vi "Send Network Message.vi"(0 "message queue in":T2, 1 "receiver process":string, 2 "receiver host":string, 3 "receiver port (0)":u16, 5 "message name":string, 7 "message value":string, 9 "timeout (25000 ms)":i32=25000, 11 "error in":errorcluster, 12 "message attributes":T1, 13 "priority message (F)":bool, 14 "acknowledge message (F)":bool) -> (4 "message queue out":T2, 10 "timed out?":bool, 15 "error out":errorcluster)   [LabVIEW 2015, in "TLB` Template.lvlib" / "AMC.lvlib"]
doc: "Adds a message to the message dispatch queue in another application instance if the receiver host and process are specified. If the receiver host and process are undefined, or if they match the local application instance, then the message is added to the appropriate local message queue.\n\nIf \"receiver port\" is undefined, this VI will attempt to use the default UDP port.\n\nIf \"priority message\" is True, the message will be added to the front of the message queue.\n\nIf \"acknowledge message\" is True and the message is sent to another application instance, the receiver will send a reply message with the name format of \"AMC_Ack\" and a value of <name>. If \"message queue in\" is undefined, no acknowledge message will be sent.TLB Prime - Application Template 1.3.0.24\nNorm Kirchner, NI Systems Engineering - NI\nCopyright (c) 2014, NI"
uses:
  AMC.lvlib
  Message Queue.ctl
  Message.ctl
  Tools/Keyed Array/KeyedArray.ctl
  Tools/Keyed Array/Tools_KeyedArray.lvlib
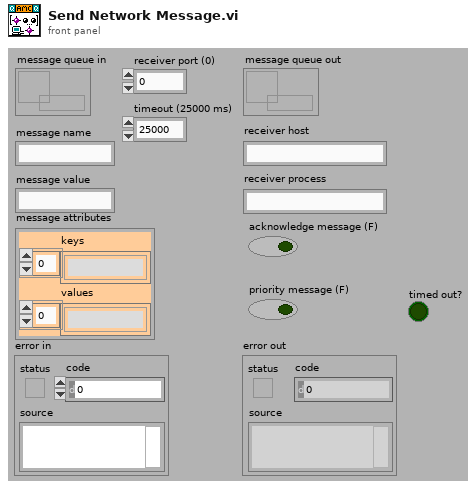
[diagram p1: front panel]
types:
  T1 = typedef "TLB` Template.lvlib/Tools_KeyedArray.lvlib/KeyedArray.ctl" = cluster{"keys":string[], "values":string[]}
  T2 = typedef "TLB` Template.lvlib/AMC.lvlib/Message Queue.ctl" = refnum<queue>
  T3 = typedef "TLB` Template.lvlib/AMC.lvlib/Message.ctl" = cluster{"name":string, "value":string, "attributes":T1, "receiver host":string, "receiver process":string, "source host":string, "source process":string, "priority message":bool, "acknowledge message":bool}
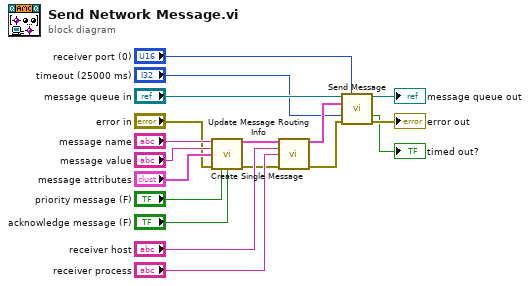
[diagram p0: block diagram]
diagram:
  n1 = call "Create Single Message.vi"("name"="message name", "value"="message value", "attributes"="message attributes", "error in"="error in", "priority message (F)"="priority message (F)", "acknowledge message (F)"="acknowledge message (F)") -> ("message"=w10:T3, "error out"=w6:errorcluster)  [unwired: 8 in]
  n2 = call "Update Message Routing Info.vi"("message"=w10, "receiver host (\"\")"="receiver host", "receiver process (\"\")"="receiver process", "error in"=w6) -> ("message"=w9:T3, "error out"=w5:errorcluster)  [unwired: 10 in]
  n3 = call "Send Message.vi"("message queue in"="message queue in", "receiver port (0)"="receiver port (0)", "message"=w9, "timeout (-1 ms)"="timeout (25000 ms)", "error in"=w5) -> ("message queue out"=→"message queue out":T2, "timed out?"=→"timed out?":bool, "error out"=→"error out":errorcluster)  [unwired: 8 in]
